vi "TS_Request Multiple Addresses.vi"(8 "error in":errorcluster, 11 "internal data":T2={"J1939 XNET Settings"={"XNET Database"="", "XNET Cluster"="", "CAN port"="", "Baud rate [Bd]"=0, "J1939 Network Address"=0, "Name"=0, "Termination"=0}, "j1939 queues"={"Processed Outgoing"=refnum, "Process Outgoing"=refnum, "stop notifier"=refnum, "error queue"=refnum, "active dtc"=refnum, "processed inc"=refnum}, "fgv references"={"BAM Buffer"=refnum, "CM Buffer"=refnum, "CM Gen"=refnum, "BAM Gen"=refnum, "Address Claims"=refnum, "RQST"=refnum, "scaling lut"=refnum, "data lut"=refnum, "cyclic scheduler"=refnum}, "frame in"="", "frame out"="", "timing"={"tb to j1939 queue timeout"=100, "j1939 to tb queue timeout"=100, "dtc loop period (ms)"=100, "CAN in loop period (ms)"=100, "process incoming queue timeout (ms)"=100, "Outgoing Write Decimation"=0, "process outgoing loop rate (ms)"=0, "periodic outgoing queue timeout (ms)"=10, "CAN out queue timeout (ms)"=100}}) -> (0 "error out":errorcluster, 2 "addresses":T1[](array[typedef]) {"Name" format="%.0x"})   [LabVIEW 2013, in "J1939.lvlib"]
uses:
  J1939.lvlib
  API Types/Internal Data.ctl
  API Types/XNET Settings.ctl
  API Types/Setup Information Cluster.ctl
  API Types/CAN Outgoing Message Cluster.ctl
  API Types/Convert DTCs Cluster.ctl
  <vilib>/xnet/xnet.llb/XNET Frame CAN.ctl
  <vilib>/xnet/xnet.llb/XNET Frame Type CAN.ctl
  TP/TP List References.ctl
  BAM/BAM Buffer Connections List_Ref.ctl
  Connection Mode/Connection Mode Generation Connection Ref.ctl
  BAM/BAM Generation Connections List_Ref.ctl
  LUTs/J1939 Address Table Reference.ctl
  RQST/RQST Lookup Table Reference.ctl
  LUTs/J1939 Conversion Lookup Table Reference.ctl
  LUTs/J1939 Data Lookup Table Reference.ctl
  LUTs/Cyclic Frame Scheduler Lut Reference.ctl
  Configuration/TypeDefs/timing configuration.ctl
  LUTs/J1939 Address Lookup Table Data.ctl
  LUTs/J1939 Address Lookup Table Action.ctl
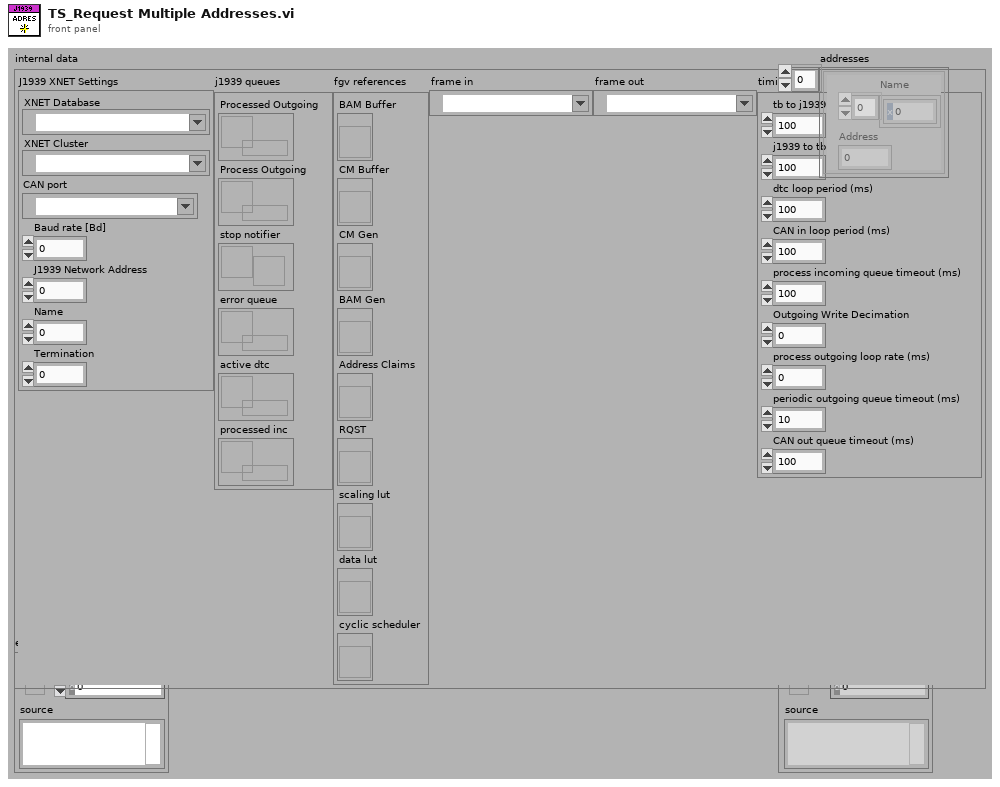
[diagram p1: front panel]
types:
  T1 = typedef "J1939.lvlib/J1939 Address Lookup Table Data.ctl" = cluster{"Name":u8[], "Address":u8}
  T2 = typedef "J1939.lvlib/Internal Data.ctl" = cluster{"J1939 XNET Settings":T3, "j1939 queues":T4, "fgv references":T5, "frame in":refnum<k21>, "frame out":refnum<k21>, "timing":T14}
  T3 = typedef "J1939.lvlib/XNET settings.ctl" = cluster{"XNET Database":refnum<k21>, "XNET Cluster":refnum<k21>, "CAN port":refnum<k21>, "Baud rate [Bd]":u32, "J1939 Network Address":u8, "Name":u64, "Termination":u32}
  T4 = typedef "J1939.lvlib/Setup Information Cluster.ctl" = cluster{"Processed Outgoing":refnum<queue>, "Process Outgoing":refnum<queue>, "stop notifier":refnum<notifier>, "error queue":refnum<queue>, "active dtc":refnum<queue>, "processed inc":refnum<queue>}
  T5 = typedef "J1939.lvlib/TP List References.ctl" = cluster{"BAM Buffer":T6, "CM Buffer":T6, "CM Gen":T7, "BAM Gen":T8, "Address Claims":T9, "RQST":T10, "scaling lut":T11, "data lut":T12, "cyclic scheduler":T13}
  T6 = typedef "J1939.lvlib/BAM Buffer Connections List_Ref.ctl" = refnum<vi>
  T7 = typedef "J1939.lvlib/Connection Mode Generation Connection Ref.ctl" = refnum<vi>
  T8 = typedef "J1939.lvlib/BAM Generation Connections List_Ref.ctl" = refnum<vi>
  T9 = typedef "J1939.lvlib/J1939 Address Table Reference.ctl" = refnum<vi>
  T10 = typedef "J1939.lvlib/RQST Lookup Table Reference.ctl" = refnum<vi>
  T11 = typedef "J1939.lvlib/J1939 Conversion Lookup Table Reference.ctl" = refnum<vi>
  T12 = typedef "J1939.lvlib/J1939 Data Lookup Table Reference.ctl" = refnum<vi>
  T13 = typedef "J1939.lvlib/cyclic frame scheduler lut reference.ctl" = refnum<vi>
  T14 = typedef "J1939.lvlib/timing configuration.ctl" = cluster{"tb to j1939 queue timeout":i32, "j1939 to tb queue timeout":i32, "dtc loop period (ms)":i32, "CAN in loop period (ms)":i32, "process incoming queue timeout (ms)":i32, "Outgoing Write Decimation":u32, "process outgoing loop rate (ms)":i32, "periodic outgoing queue timeout (ms)":i32, "CAN out queue timeout (ms)":i32}
  T15 = typedef "J1939.lvlib/J1939 Address Lookup Table Action.ctl" = enum16{"Initialize", "Add", "Get", "Remove", "Get All"}
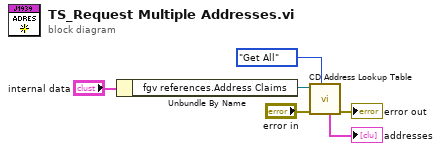
[diagram p0: block diagram]
diagram:
  n1 = Unbundle By Name("internal data") -> ("fgv references.Address Claims"=w3:T9)
  n2 = call "CD Address Lookup Table.vi"("Action"=J1939_Address_Lookup_Table_Action."Get All", "error in (no error)"="error in", "ref in"=w3) -> ("error out"=→"error out":errorcluster, "All Data"=→"addresses":T1[])  [unwired: 5 in, 2 out]
